vi "GVISA Mux Close.vi"(8 "error in":errorcluster, 11 "session in":T1={"VISA"="", "paths"=[], "idn command"="", "serial cfg"={"Baud rate"=9600, "Data bits"=8, "Parity"=0, "Stop bits"=10, "Flow control"=0, "End Mode Read"=enum."None", "End Mode Write"=enum."None", "Term character"=0, "Term enable"=FALSE}} {"serial cfg"."Flow control" items=["None", "XON/XOFF", "CTS/RTS", "XON/XOFF + CTS/RTS", "DTR/DSR", "XON/XOFF + DTR/DSR"]; "serial cfg"."Stop bits" items=["1 bit"=10, "1.5 bits"=15, "2 bits"=20]; "serial cfg"."Parity" items=["None", "Odd", "Even", "Mark", "Space"]; "serial cfg"."Data bits" items=["5 bits"=5, "6 bits"=6, "7 bits"=7, "8 bits"=8]; "serial cfg"."Baud rate" items=["150 Bd"=150, "300 Bd"=300, "600 Bd"=600, "1200 Bd"=1200, "2400 Bd"=2400, "4800 Bd"=4800, "9600 Bd"=9600, "19.2 kBd"=19200, "38.4 kBd"=38400, "57.6 kBd"=57600, "115.2 kBd"=115200]}) -> (0 "error out":errorcluster, 3 "session out":T1={"VISA"="", "paths"=[], "idn command"="", "serial cfg"={"Baud rate"=9600, "Data bits"=8, "Parity"=0, "Stop bits"=10, "Flow control"=0, "End Mode Read"=enum."None", "End Mode Write"=enum."None", "Term character"=0, "Term enable"=FALSE}} {"serial cfg"."Flow control" items=["None", "XON/XOFF", "CTS/RTS", "XON/XOFF + CTS/RTS", "DTR/DSR", "XON/XOFF + DTR/DSR"]; "serial cfg"."Stop bits" items=["1 bit"=10, "1.5 bits"=15, "2 bits"=20]; "serial cfg"."Parity" items=["None", "Odd", "Even", "Mark", "Space"]; "serial cfg"."Data bits" items=["5 bits"=5, "6 bits"=6, "7 bits"=7, "8 bits"=8]; "serial cfg"."Baud rate" items=["150 Bd"=150, "300 Bd"=300, "600 Bd"=600, "1200 Bd"=1200, "2400 Bd"=2400, "4800 Bd"=4800, "9600 Bd"=9600, "19.2 kBd"=19200, "38.4 kBd"=38400, "57.6 kBd"=57600, "115.2 kBd"=115200]})   [LabVIEW 2020]
doc: "Close generic VISA command mutiplexer session."
uses:
  GVISA Mux Session.ctl
  GVISA Mux Path Entry.ctl
  met_serial_setup.ctl
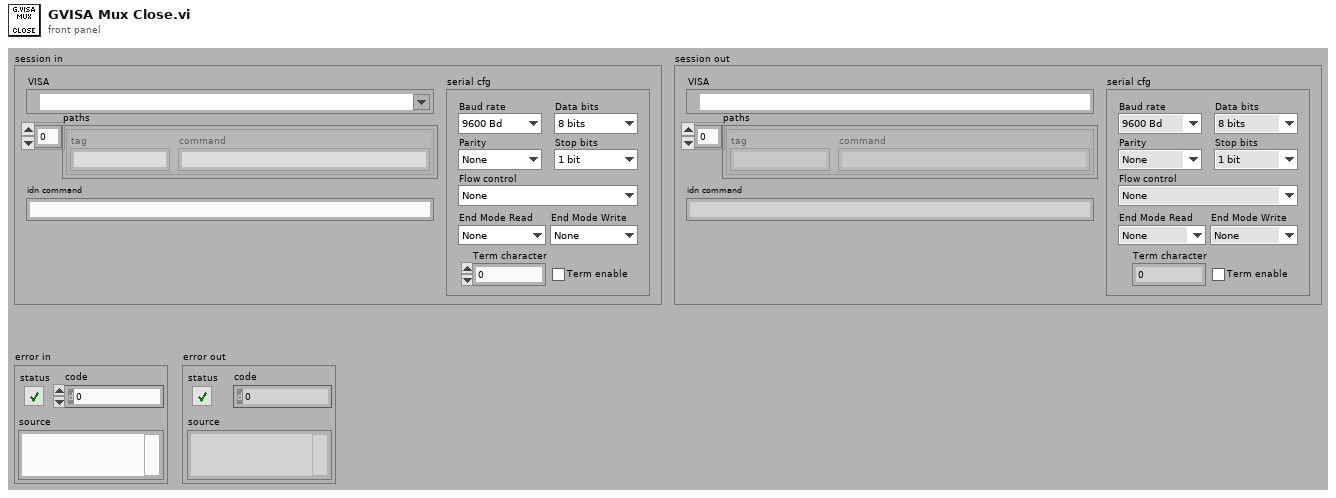
[diagram p1: front panel]
types:
  T1 = typedef "GVISA Mux Session.ctl" = cluster{"VISA":refnum<visa-resource-name>, "paths":T2[], "idn command":string, "serial cfg":T3}
  T2 = typedef "GVISA Mux Path Entry.ctl" = cluster{"tag":string, "command":string}
  T3 = typedef "met_serial_setup.ctl" = cluster{"Baud rate":i32, "Data bits":i32, "Parity":i32, "Stop bits":i32, "Flow control":i32, "End Mode Read":enum16{"None", "Last Bit", "TermChar"}, "End Mode Write":enum16{"None", "Last Bit", "TermChar"}, "Term character":u8, "Term enable":bool}
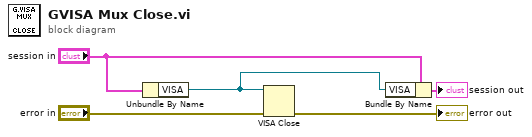
[diagram p0: block diagram]
diagram:
  n1 = Unbundle By Name("session in") -> ("VISA"=w1:refnum<visa-resource-name>)
  n2 = VISA Close(VISA resource name=w1, error in (no error)="error in") -> (error out=→"error out":errorcluster)
  n3 = Bundle By Name(cluster="session in", "VISA"=w1) -> (→"session out":T1)
